vi "calcForceError.vi"(8 "error in (no error)":errorcluster, 11 "SystemController in":refnum<class "SystemController.lvclass">) -> (0 "error out":errorcluster, 1 "Force Error":T1 min=-888.0 max=888.0 format="%.2f", 2 "Force Demand":T1 min=-888.0 max=888.0 format="%.2f", 3 "SystemController out":refnum<class "SystemController.lvclass">)   [LabVIEW 2013, in "SystemController.lvclass"]
uses:
  SystemController.lvclass
  Typedefs/ForceDemand.ctl
  SystemController.lvclass/SystemController.ctl
  Typedefs/M2AADTTypedefs.lvlib
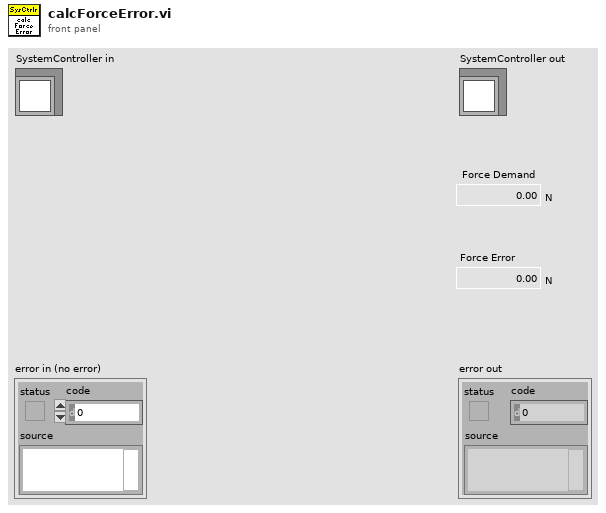
[diagram p1: front panel]
types:
  T1 = typedef "M2AADTTypedefs.lvlib/ForceDemand.ctl" = dbl[unit]
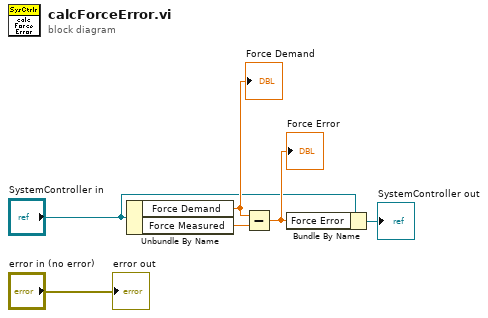
[diagram p0: block diagram]
diagram:
  n1 = Unbundle By Name("SystemController in") -> ("Force Demand"=w5:T1, "Force Measured"=w1:T1)
  "Force Demand" <- w5
  n2 = Subtract(x=w5, y=w1) -> (x-y=w4:T1)
  "Force Error" <- w4
  n3 = Bundle By Name(cluster="SystemController in", "Force Error"=w4) -> (→"SystemController out":refnum<class "SystemController.lvclass">)
  "error out" <- "error in (no error)"
